vi "Valve-Pulse.vi"(7 "Device reference":refnum<vi>, 8 "error in (no error)":errorcluster, 9 "Eventstring":string="auto-generate", 10 "Duration":i32) -> (0 "error out":errorcluster, 2 "Actual duration":i32)   [LabVIEW 2015]
doc: "Pulses a juicer valve.\n\nDevice reference: which valve?\nDuration: how long to open for?\n--positive: specifies open duration in ms\n--unwired or 0: accept default from valve ref.\n--negative: open indefinitely\nEventstring: used for timestamping\n--empty: no timestamp will be generated\n--unwired or \"auto-generate\": TS w/ default eventstring\n--otherwise: TS with user-provided string\nAcutal duration: the actual commanded pulse duration. Useful if you decided to use the default value.\n\nThe default eventstring is:\n[valve name].open.[duration]\nwhere [valve name] is the referenced valve's front panel label text and [duration] will have the actual duration filled in if the Duration input was left unwired (or set to 0)."
uses:
  Typedefs/Valve.ctl
  Rack/Typedefs/OutputRequest refnum.ctl
  Rack/Typedefs/OutputRequest.ctl
  Rack/Typedefs/InputData cluster.ctl
  Rack/Methods/Port drivers/DigitalInput-DataCluster.ctl
panel:
  # "(must be on same NI card)"
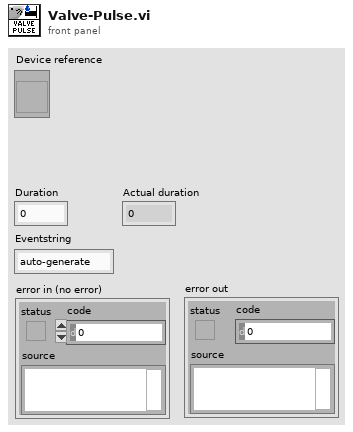
[diagram p1: front panel]
types:
  T1 = typedef "Valve.ctl" = cluster{"Settings":cluster{"Timestamp port name":string, "Port name":string, "Port index":i32}, "OutputRequest event ref":T2, "InputData reference":refnum<vi>, "Default length (ms)":i32}
  T2 = typedef "OutputRequest refnum.ctl" = refnum<user-event>
  T3 = typedef "OutputRequest.ctl" = cluster{"Target":string, "Command":string}
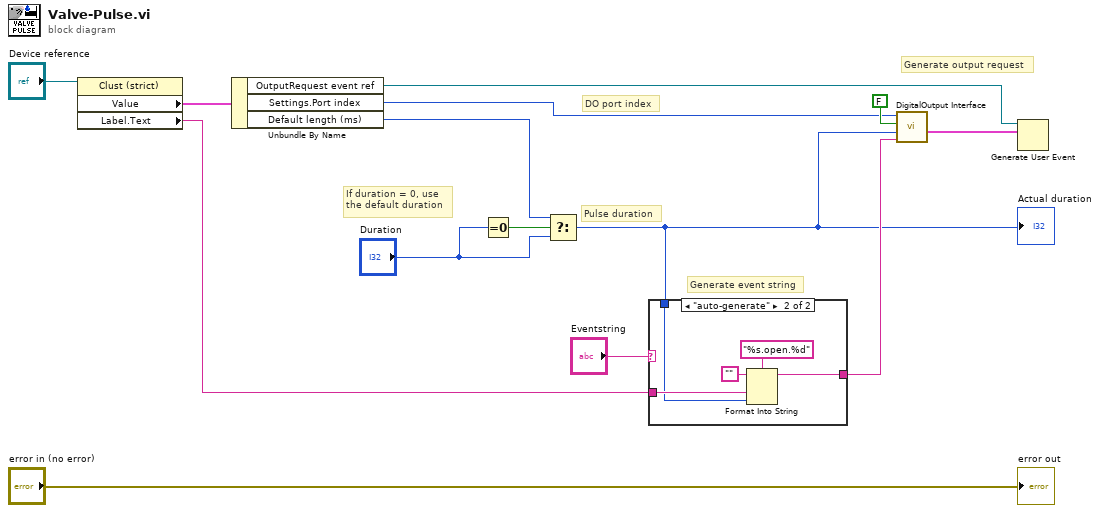
[diagram p0: block diagram]
diagram:
  # "Pulse duration"
  # "DO port index"
  # "Generate output request"
  # "Generate event string"
  # "If duration = 0, use \nthe default duration"
  n1 = property class="Clust (strict)"(reference="Device reference") -> ("Value"=w14:T1, "Label.Text"=w9:string)  [unwired: 1 in, 2 out]
  n2 = Unbundle By Name(w14) -> ("OutputRequest event ref"=w4:T2, "Settings.Port index"=w2:i32, "Default length (ms)"=w1:i32)
  n3 = Equal To 0?(x="Duration") -> (x = 0?=w11:bool)
  n4 = Select(t=w1, s=w11, f="Duration") -> (s? t:f=w5:i32)
  "Actual duration" <- w5
  n5 = case shown="\"auto-generate\"" "Eventstring" {
    selector: "Eventstring" -> [w15 _]
    tunnel: w9 -> [_ w18]
    tunnel: [w15 w17] -> w7
    tunnel: w5 -> [_ w16]
    frame Default {
      # "Use user-provided string"
    }
    frame "auto-generate" {
      n6 = Format Into String(format string="%s.open.%d", initial string="", w18, w16) -> (resulting string=w17:string)  [unwired: 1 in, 1 out]
    }
  }
  n7 = call "DigitalOutput Interface.vi"("Eventstring"=w7, "Pulse duration (-1 for cont.)"=w5, "On/off"=FALSE, "Port index"=w2) -> ("OutputRequest"=w6:T3)  [unwired: 7 in]
  n8 = Generate User Event(user event=w4, event data cluster=w6) -> ()  [unwired: 2 in, 2 out]
  "error out" <- "error in (no error)"
